vi "Evaluate with new Params.vi"(8 "error in (no error)":errorcluster, 11 "HIJ Vision Display in":refnum<class "HIJ Vision Display.lvclass">) -> (0 "error out":errorcluster, 3 "HIJ Vision Display out":refnum<class "HIJ Vision Display.lvclass">)   [LabVIEW 2014, in "HIJ Vision Display.lvlib" / "HIJ Vision Display.lvclass"]
uses:
  HIJ Vision Display.lvclass
  HIJ Vision Display.lvclass/HIJ Vision Display.ctl
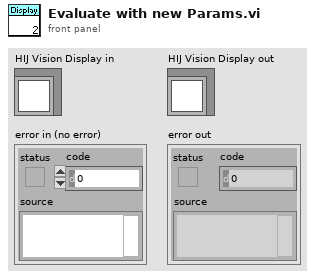
[diagram p1: front panel]
types:
  T1 = typedef "IMAQ Image.ctl" = refnum<image>
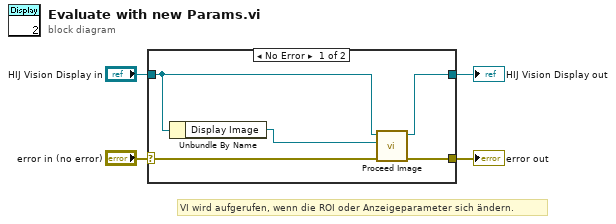
[diagram p0: block diagram]
diagram:
  # "VI wird aufgerufen, wenn die ROI oder Anzeigeparameter sich ändern."
  n1 = case shown="No Error" "error in (no error)" {
    selector: "error in (no error)" -> [w7 w11]
    tunnel: [w6 w11] -> w3
    tunnel: [w9 w10] -> w1
    tunnel: "HIJ Vision Display in" -> [w8 w10]
    frame No Error {
      n2 = Unbundle By Name(w8) -> ("Display Image"=w5:T1)
      n3 = call "Proceed Image.vi"("error in (no error)"=w7, "Image"=w5, "IMAQ Display in"=w8) -> ("error out"=w6:errorcluster, "HIJ Vision Display out"=w9:refnum<class "HIJ Vision Display.lvclass">)  [unwired: 7 in]
    }
    frame Error {
    }
  }
  "error out" <- w3
  "HIJ Vision Display out" <- w1
